vi "Tool Q LEIN stroke Go To.vi"(1 "Retry on err (F)":bool, 5 "current limit(0.2A)":dbl, 7 "Target positio pulses":dbl, 9 "time (50 ms)":u16, 11 "error in (no error)":errorcluster) -> (4 "LEIN custom reply Q":T1, 15 "error out":errorcluster)   [LabVIEW 2011]
uses:
  LEINmaster/Defenitions/LEIN custom reply Q.ctl
  LEINmaster/Defenitions/LEIN Reply Holder.ctl
  LEINmaster/Defenitions/LEIN CMD Cluster.ctl
  LEINmaster/Defenitions/LEIN CMD List.ctl
  LEINmaster/Defenitions/LEIN Structure variations.ctl
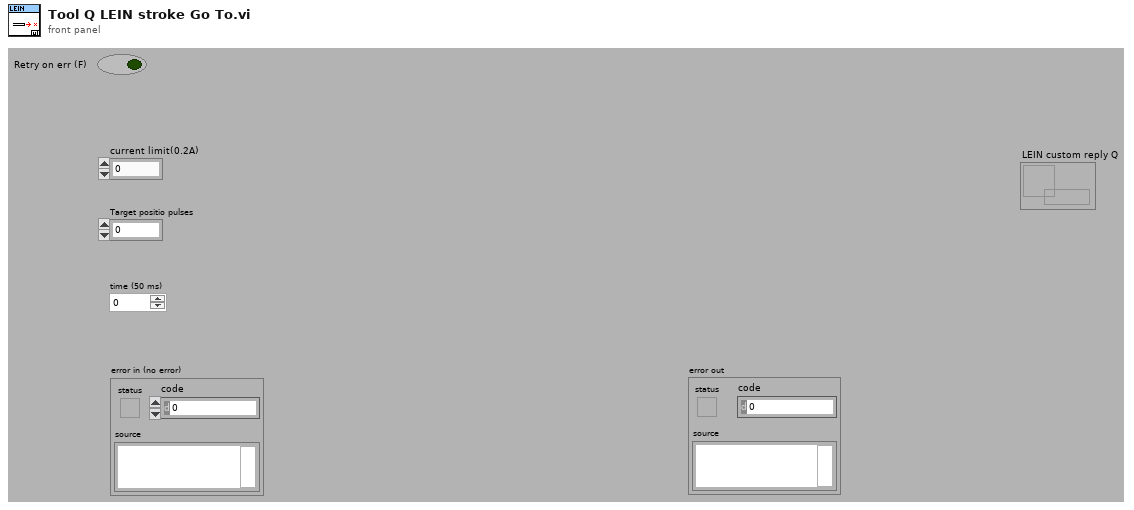
[diagram p1: front panel]
types:
  T1 = typedef "LEIN custom reply Q.ctl" = refnum<queue>
  T2 = typedef "LEIN Structure variations.ctl" = enum16{"LEIN08", "LEIN31", "LEIN63"}
  T3 = enum16{"big-endian, network order", "native, host order", "little-endian"}
  T4 = typedef "LEIN CMD Cluster.ctl" = cluster{"SID":u8, "ANF":bool, "CMD":T5, "DATA":u8[]}
  T5 = typedef "LEIN CMD List.ctl" = enum8{"ACTI", "TASK", "RES0", "STAT", "RES1", "RES2", "RES3", "USER"}
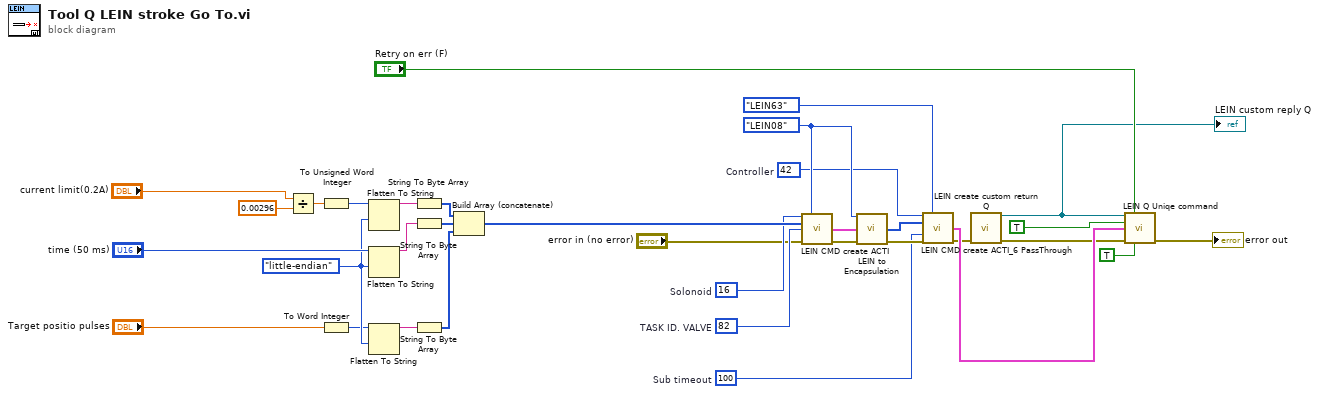
[diagram p0: block diagram]
diagram:
  w14 = u8 42  # Controller
  w15 = u8 16  # Solonoid
  w21 = u16 100  # Sub timeout
  w18 = u8 82  # TASK ID. VALVE
  w17 = LEIN_Structure_variations."LEIN08" ("LEIN Variation")
  w10 = T3."little-endian" ("byte order (0:big-endian, network order)")
  n1 = Divide(x="current limit(0.2A)", y=0.00296 ("x")) -> (x/y=w33:dbl)
  n2 = To Unsigned Word Integer(number=w33) -> (unsigned 16bit integer=w31:u16)
  n3 = To Word Integer(number="Target positio pulses") -> (16bit integer=w9:i16)
  n4 = Flatten To String(anything=w31, byte order (0:big-endian, network order)=w10) -> (data string=w30:string)  [unwired: 2 in, 2 out]
  n5 = Flatten To String(anything="time (50 ms)", byte order (0:big-endian, network order)=w10) -> (data string=w27:string)  [unwired: 2 in, 2 out]
  n6 = Flatten To String(anything=w9, byte order (0:big-endian, network order)=w10) -> (data string=w8:string)  [unwired: 2 in, 2 out]
  n7 = String To Byte Array(string=w30) -> (unsigned byte array=w29:u8[])
  n8 = String To Byte Array(string=w27) -> (unsigned byte array=w26:u8[])
  n9 = String To Byte Array(string=w8) -> (unsigned byte array=w7:u8[])
  n10 = Build Array (concatenate)(w29, w26, w7) -> (w16:u8[])
  n11 = call "LEIN CMD create ACTI.vi"("SID"=w15, "LEIN Variation"=w17, "Data"=w16, "ACTI ID"=w18, "error in (no error)"="error in (no error)") -> ("CMD"=w19:T4, "error out"=w20:errorcluster)  [unwired: 9 in]
  n12 = call "LEIN to Encapsulation.vi"("LEIN Variation"=w17, "CMD"=w19, "error in (no error)"=w20) -> ("Data and header"=w22:u8[], "error out"=w23:errorcluster)  [unwired: 8 in, 3 out]
  n13 = call "LEIN CMD create ACTI_6 PassThrough.vi"("SID"=w14, "LEIN Variation"=LEIN_Structure_variations."LEIN63", "LEIN ecapsulated data (header and data)"=w22, "Sub Timeout (ms)"=w21, "error in (no error)"=w23) -> ("CMD"=w6:T4, "error out"=w5:errorcluster)  [unwired: 9 in]
  n14 = call "LEIN create custom return Q.vi"("error in (no error)"=w5) -> ("LEIN custom reply Q"=w4:T1, "error out"=w2:errorcluster)  [unwired: 13 in]
  "LEIN custom reply Q" <- w4
  n15 = call "LEIN Q Uniqe command.vi"("LEIN custom reply Q"=w4, "Retry on err (F)"="Retry on err (F)", "Custom Q(F)"=TRUE, "CMD"=w6, "error in"=w2, "priority(F)"=TRUE) -> ("error out"=→"error out":errorcluster)  [unwired: 9 in]
